vi "Configure NRPM Measurement.vi"(6 "Repetition (Single)":i32(ring) items=["Single", "Continuous"], 7 "Statistic Count (1)":i32=1, 8 "error in (no error)":errorcluster, 9 "Measurement Timeout (1)":dbl=1.0 format="%^.3e", 10 "Instance (1)":i32=1, 11 "VISA resource name":refnum<visa-resource-name>) -> (0 "error out":errorcluster, 3 "VISA resource name out":refnum<visa-resource-name>)   [LabVIEW 2020, in "Rohde&Schwarz CMXP GPRF.lvlib"]
doc: "Configures the NRPM Measurement.\n\nAttributes:\nRSCMXPGPRF_ATTR_NRPM_MEASUREMENT_TIMEOUT\nRSCMXPGPRF_ATTR_NRPM_MEASUREMENT_STATISTIC_COUNT\nRSCMXPGPRF_ATTR_NRPM_MEASUREMENT_REPETITION\n\nRemote-control commands:\nCONFigure:GPRF:MEAS<i>:NRPM:TOUT\nCONFigure:GPRF:MEAS<i>:NRPM:SCOunt\nCONFigure:GPRF:MEAS<i>:NRPM:REPetition"
uses:
  <instrlib>/Rohde&Schwarz CMXP GPRF/Rohde&Schwarz CMXP GPRF.lvlib
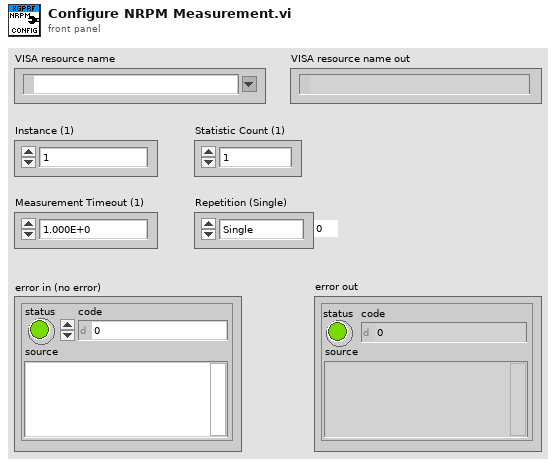
[diagram p1: front panel]
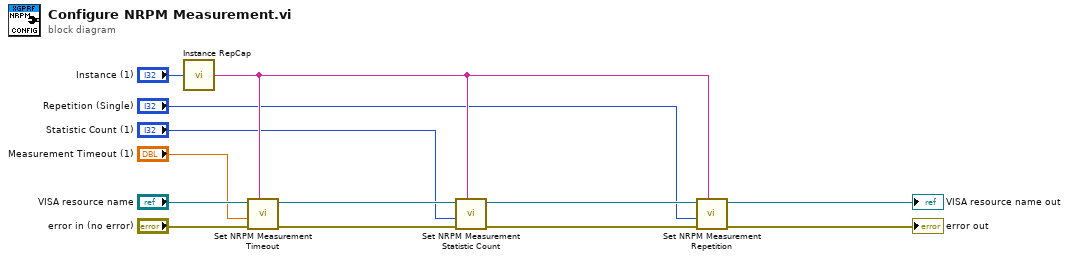
[diagram p0: block diagram]
diagram:
  n1 = call <instrlib>:"Instance RepCap.vi"("Instance in"="Instance (1)") -> ("Instance out"=w4:string)
  n2 = call "Set NRPM Measurement Timeout"("Repeated Capabilities"=w4, "error in (no error)"="error in (no error)", "NRPM Measurement Timeout (0.0)"="Measurement Timeout (1)", "instrument handle"="VISA resource name") -> ("error out"=w10:errorcluster, "instrument handle out"=w11:refnum<visa-resource-name>)  [unwired: 6 in]
  n3 = call "Set NRPM Measurement Statistic Count"("Repeated Capabilities"=w4, "error in (no error)"=w10, "NRPM Measurement Statistic Count (0)"="Statistic Count (1)", "instrument handle"=w11) -> ("error out"=w6:errorcluster, "instrument handle out"=w7:refnum<visa-resource-name>)  [unwired: 6 in]
  n4 = call "Set NRPM Measurement Repetition"("Repeated Capabilities"=w4, "error in (no error)"=w6, "NRPM Measurement Repetition (0 - Single)"="Repetition (Single)", "instrument handle"=w7) -> ("error out"=→"error out":errorcluster, "instrument handle out"=→"VISA resource name out":refnum<visa-resource-name>)  [unwired: 6 in]
